vi "Set XY.vi"(0 "reference in":refnum<class "Operation.lvclass">, 1 "x":dbl, 3 "y":dbl, 5 "error in (no error)":errorcluster) -> (14 "reference out":refnum<class "Operation.lvclass">, 19 "error out":errorcluster)   [LabVIEW 2013, in "Operation.lvclass"]
uses:
  Operation.lvclass
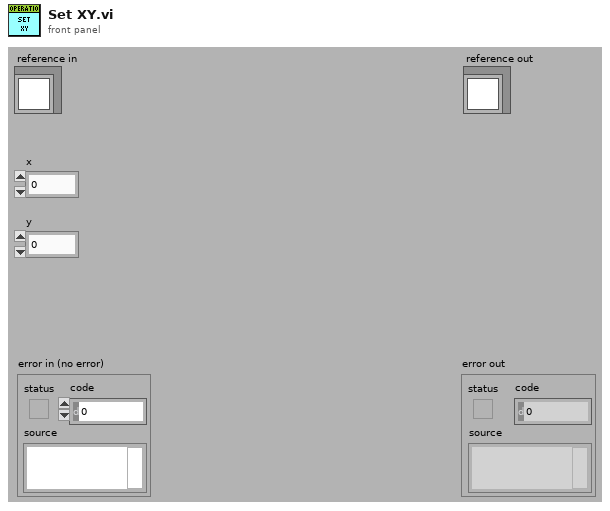
[diagram p1: front panel]
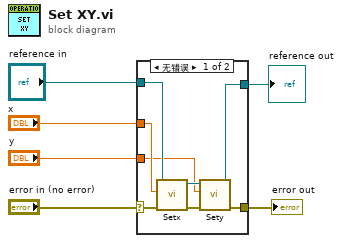
[diagram p0: block diagram]
diagram:
  n1 = case shown="无错误" "error in (no error)" {
    selector: "error in (no error)" -> [w11 w16]
    tunnel: [w9 w16] -> w5
    tunnel: [w12 w15] -> w3
    tunnel: "reference in" -> [w14 w15]
    tunnel: "x" -> [w8 _]
    tunnel: "y" -> [w7 _]
    frame No Error {
      n2 = call "Setx.vi"("error in (no error)"=w11, "x"=w8, "reference in"=w14) -> ("error out"=w10:errorcluster, "reference out"=w13:refnum<class "Operation.lvclass">)  [unwired: 7 in]
      n3 = call "Sety.vi"("error in (no error)"=w10, "y"=w7, "reference in"=w13) -> ("error out"=w9:errorcluster, "reference out"=w12:refnum<class "Operation.lvclass">)  [unwired: 7 in]
    }
    frame Error {
    }
  }
  "error out" <- w5
  "reference out" <- w3
